vi "Scale and Mean.vi"(10 "Slope & Offset":sgl[][](array[numeric]), 11 "Raw In":sgl[][](array[numeric])) -> (1 "RAW Mean":sgl[](array[numeric]), 2 "Scaled Value":sgl[][](array[numeric]), 3 "Scaled Mean":sgl[](array[numeric]))   [LabVIEW 2018]
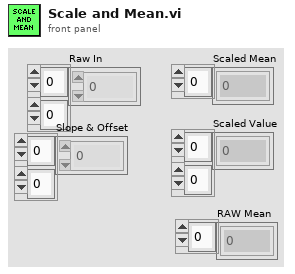
[diagram p1: front panel]
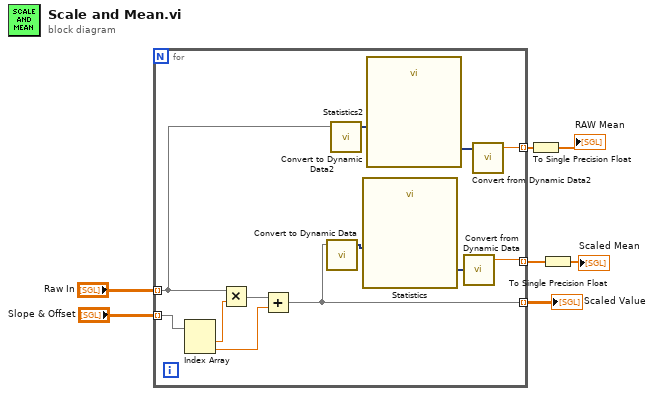
[diagram p0: block diagram]
diagram:
  n1 = for {
    tunnel: "Raw In" -> [w11] mode=indexing
    tunnel: [w12] -> w7 mode=indexing
    tunnel: [w17] -> w6 mode=indexing
    tunnel: "Slope & Offset" -> [w16] mode=indexing
    tunnel: [w8] -> w2 mode=indexing
    n2 = Index Array(array=w16) -> (element #1=w15:sgl, element #2=w13:sgl)  [unwired: 2 in]
    n3 = Multiply(x=w11, y=w15) -> (x*y=w14:sgl[])
    n4 = Add(x=w14, y=w13) -> (x+y=w12:sgl[])
    n5 = call "Convert to Dynamic Data"("Array"=w12) -> ("Dynamic Data Type"=w19:dynamicdata)  [unwired: 3 in]
    n6 = call "Convert to Dynamic Data2"("Array"=w11) -> ("Dynamic Data Type"=w10:dynamicdata)  [unwired: 3 in]
    n7 = call "Statistics"("Signals"=w19) -> ("Arithmetic Mean"=w18:dynamicdata)  [unwired: 25 in, 1 out]
    n8 = call "Statistics2"("Signals"=w10) -> ("Arithmetic Mean"=w9:dynamicdata)  [unwired: 25 in, 1 out]
    n9 = call "Convert from Dynamic Data"("Dynamic Data Type"=w18) -> ("Scalar"=w17:dbl)  [unwired: 3 in]
    n10 = call "Convert from Dynamic Data2"("Dynamic Data Type"=w9) -> ("Scalar"=w8:dbl)  [unwired: 3 in]
  }
  "Scaled Value" <- w7
  n11 = To Single Precision Float(number=w2) -> (single precision float=→"RAW Mean":sgl[])
  n12 = To Single Precision Float(number=w6) -> (single precision float=→"Scaled Mean":sgl[])
